vi "Read Best Solution Array.vi"(8 "error in (no error)":errorcluster, 11 "GA in":refnum<class "GA.lvclass">) -> (0 "error out":errorcluster, 2 "Best Solution Array":T1[](array[typedef]), 3 "GA out":refnum<class "GA.lvclass">)   [LabVIEW 2013, in "GA.lvclass"]
uses:
  GA.lvclass
  Controls/Solution.ctl
  GA.lvclass/GA.ctl
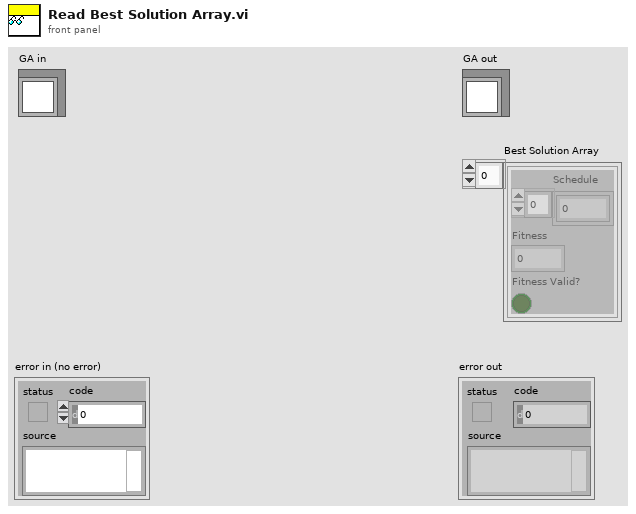
[diagram p1: front panel]
types:
  T1 = typedef "Solution.ctl" = cluster{"Schedule":u16[], "Fitness":u16, "Fitness Valid?":bool}
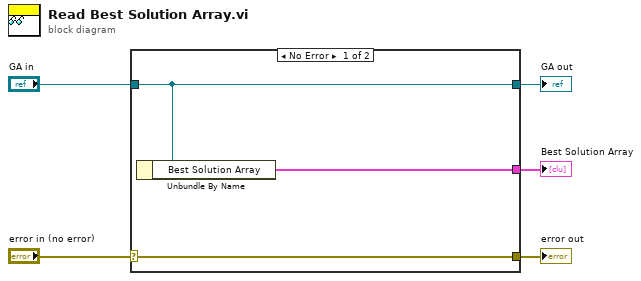
[diagram p0: block diagram]
diagram:
  n1 = case shown="No Error" "error in (no error)" {
    selector: "error in (no error)" -> [w8 w9]
    tunnel: [w8 w9] -> w4
    tunnel: [w7 w10] -> w2
    tunnel: "GA in" -> [w7 w10]
    tunnel: [w6 _] -> w1
    frame No Error {
      n2 = Unbundle By Name(w7) -> ("Best Solution Array"=w6:T1[])
    }
    frame Error {
    }
  }
  "error out" <- w4
  "GA out" <- w2
  "Best Solution Array" <- w1
